vi "Conversion.vi"(5 "Input = DBL/String (DBL[false])":bool, 6 "Microsteps (MS=64)":dbl=64.0, 7 "Motor":u16(ring)=3 items=["none", "1", "2", "3", "4", "all"], 8 "Output Unit":T1=enum."Angle [TMC]", 9 "Input Unit":T1=enum."Inches", 10 "Input String":string="0", 11 "Input":dbl format="%#_13g") -> (2 "Output":string="0", 3 "Output DBL":dbl)   [LabVIEW 2013]
uses:
  Unit_Control.ctl
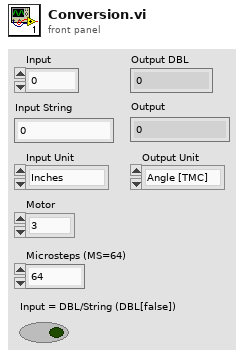
[diagram p1: front panel]
types:
  T1 = typedef "Unit_Control.ctl" = enum16{"Angle (Degrees)", "Rad", "Angle [TMC]", "Microsteps [TMC]", "Inches", "Nanometer", "Meter", "Centimeter", "Millimeter", "Micron", "Joule", "Electron Volts", "Hertz", "Terahertz", "Megahertz"}
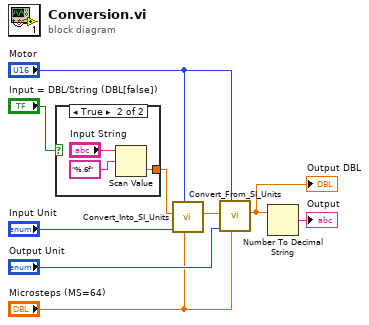
[diagram p0: block diagram]
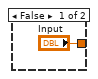
[diagram p2: hidden frame]
diagram:
  n1 = case shown="True" "Input = DBL/String (DBL[false])" {
    tunnel: ["Input" w11] -> w3
    frame False {
    }
    frame True {
      n2 = Scan Value(string="Input String", format string="%.6f") -> (value=w11:dbl)  [unwired: 1 in, 1 out]
    }
  }
  n3 = call "Convert_Into_SI_Units.vi"("Microsteps (MS=64)"="Microsteps (MS=64)", "Motor"="Motor", "Input Unit"="Input Unit", "Input"=w3) -> ("Output"=w8:dbl)  [unwired: 7 in]
  n4 = call "Convert_From_SI_Units.vi"("Microsteps (MS=64)"="Microsteps (MS=64)", "Motor"="Motor", "Output Unit"="Output Unit", "Input"=w8) -> ("Output"=w2:dbl)  [unwired: 7 in]
  "Output DBL" <- w2
  n5 = Number To Decimal String(number=w2) -> (decimal integer string=→"Output":string)  [unwired: 1 in]
